vi "CMD_ERROR.vi"(6 "Gantry in":refnum<class "Gantry.lvclass">, 8 "error in (no error)":errorcluster, 10 "Arguments":string[](array[string]), 11 "gScript Interpreter in":refnum<class "gScript Interpreter.lvclass">) -> (0 "error out":errorcluster, 3 "gScript Interpreter out":refnum<class "gScript Interpreter.lvclass">, 4 "Gantry out":refnum<class "Gantry.lvclass">)   [LabVIEW 2024, in "gScript Interpreter.lvclass"]
uses:
  gScript Interpreter.lvclass
  Shared Components/Gantry Class/Gantry.lvclass
  gScript Interpreter.lvclass/gScript Interpreter.ctl
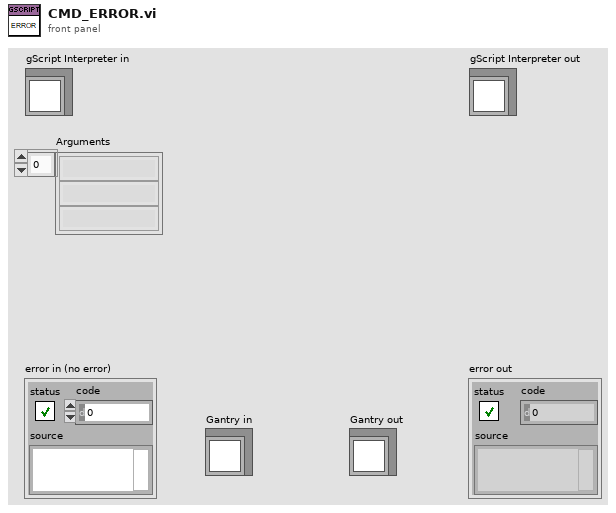
[diagram p1: front panel]
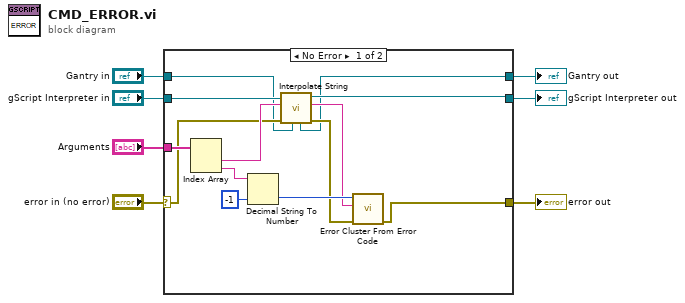
[diagram p0: block diagram]
diagram:
  n1 = case shown="No Error" "error in (no error)" {
    selector: "error in (no error)" -> [w12 w23]
    tunnel: [w16 w23] -> w4
    tunnel: [w10 w22] -> w3
    tunnel: "gScript Interpreter in" -> [w15 w22]
    tunnel: "Arguments" -> [w20 _]
    tunnel: "Gantry in" -> [w9 w21]
    tunnel: [w8 w21] -> w1
    frame No Error {
      n2 = Index Array(array=w20) -> (element #1=w14:string, element #2=w19:string)  [unwired: 2 in]
      n3 = Decimal String To Number(string=w19, default (0L)=-1 ("default (0 I32)")) -> (number=w17:i32)  [unwired: 1 in, 1 out]
      n4 = call-dynamic "Interpolate String.vi"("Gantry in"=w9, "error in (no error)"=w12, "Input String"=w14, "gScript Interpreter in"=w15) -> ("error out"=w11:errorcluster, "Output String"=w13:string, "gScript Interpreter out"=w10:refnum<class "gScript Interpreter.lvclass">, "Gantry out"=w8:refnum<class "Gantry.lvclass">)  [unwired: 4 in]
      n5 = call <vilib>:"Error Cluster From Error Code.vi"("error in (no error)"=w11, "error message (\"\")"=w13, "error code (0)"=w17) -> ("error out"=w16:errorcluster)  [unwired: 6 in]
    }
    frame Error {
    }
  }
  "error out" <- w4
  "gScript Interpreter out" <- w3
  "Gantry out" <- w1
